vi "Append Source Name.vi"(6 "Log Packet":T1, 11 "Network Sink in":refnum<class "Network Sink.lvclass">) -> (3 "Network Sink out":refnum<class "Network Sink.lvclass">, 4 "Log Packet  Out":T1)   [LabVIEW 2017, in "Network Sink.lvlib" / "Network Sink.lvclass"]
uses:
  <vilib>/gpm_packages/@cs/event-logger/Source/Network Sink/Network Sink/Network Sink.lvclass
  <vilib>/gpm_packages/@cs/event-logger/Source/Composed Log/Types/Log Packet.ctl
  <vilib>/gpm_packages/@cs/event-logger/Source/Composed Log/Types/Log Level.ctl
  <vilib>/gpm_packages/@cs/event-logger/Source/Network Sink/Network Sink/Network Sink.lvclass/Network Sink.ctl
  <vilib>/gpm_packages/@cs/event-logger/Source/Composed Log/Composed Log.lvlib
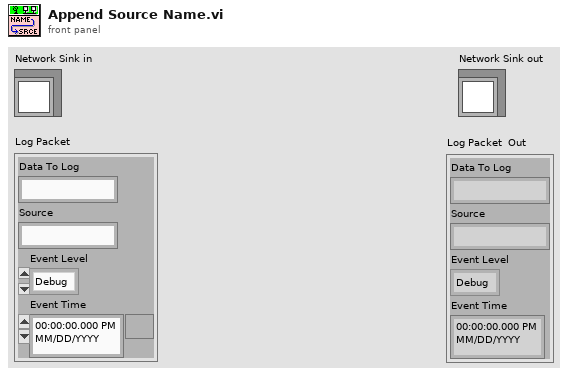
[diagram p1: front panel]
types:
  T1 = typedef "Composed Log.lvlib/Log Packet.ctl" = cluster{"Data To Log":string, "Source":string, "Event Level":T2, "Event Time":timestamp}
  T2 = typedef "Composed Log.lvlib/Log Level.ctl" = enum16{"Debug", "Info", "Warning", "Error", "Critical"}
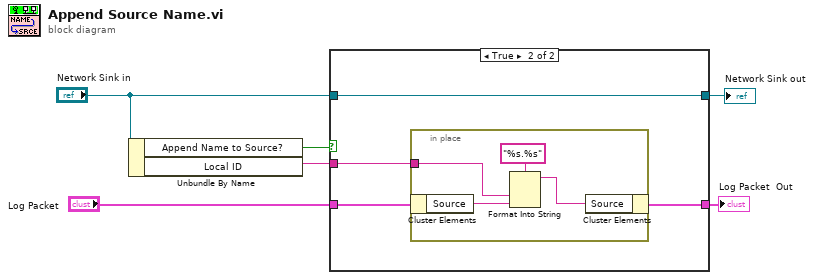
[diagram p0: block diagram]
diagram:
  n1 = Unbundle By Name("Network Sink in") -> ("Append Name to Source?"=w1:bool, "Local ID"=w2:string)
  n2 = case shown="True" w1 {
    tunnel: "Log Packet" -> [w7 w12]
    tunnel: "Network Sink in" -> [w8 w10]
    tunnel: [w8 w10] -> w5
    tunnel: [w7 w11] -> w3
    tunnel: w2 -> [_ w9]
    frame False {
    }
    frame True {
      n3 = in-place {
        in-place-border: w9 -> [w15]
        n4 = in-place-cluster #1(w12) -> ("Source"=w16:string)
        n5 = Format Into String(format string="%s.%s", w15, w16) -> (resulting string=w13:string)  [unwired: 2 in, 1 out]
        n6 = in-place-cluster #1("Source"=w13) -> (w11:T1)
      }
    }
  }
  "Network Sink out" <- w5
  "Log Packet  Out" <- w3
